vi "Merge.vi"(6 "Conditional Object":refnum<class>, 8 "error in (no error)":errorcluster, 9 "Object B":refnum<class>, 10 "Object A":refnum<class>, 11 "Overwrite A if A equal in":refnum<class "Overwrite A if A equal.lvclass">) -> (0 "error out":errorcluster, 2 "Output Object":refnum<class>, 3 "Overwrite A if A equal out":refnum<class "Overwrite A if A equal.lvclass">)   [LabVIEW 2020, in "Merge Tools.lvlib" / "Overwrite A if A equal.lvclass"]
uses:
  Overwrite A if A equal.lvclass
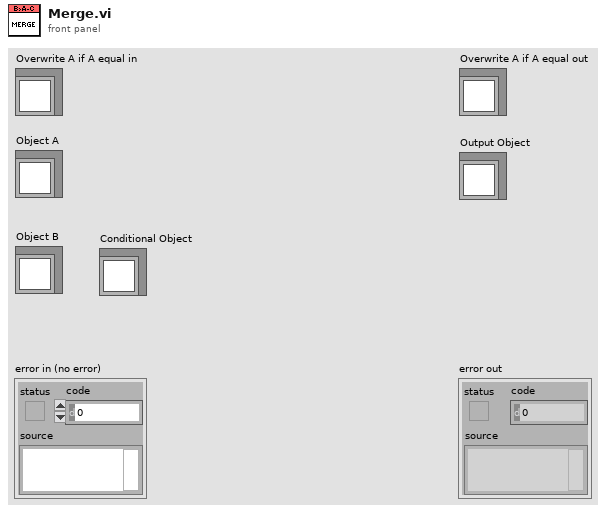
[diagram p1: front panel]
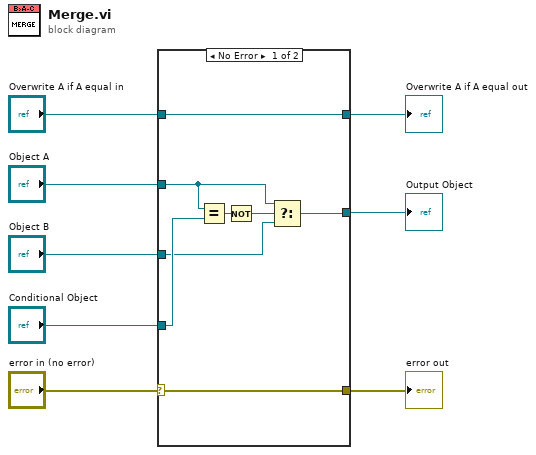
[diagram p0: block diagram]
diagram:
  n1 = case shown="No Error" "error in (no error)" {
    selector: "error in (no error)" -> [w9 w18]
    tunnel: [w9 w18] -> w7
    tunnel: "Overwrite A if A equal in" -> [w10 w17]
    tunnel: [w10 w17] -> w5
    tunnel: "Object A" -> [w13 _]
    tunnel: "Object B" -> [w12 _]
    tunnel: "Conditional Object" -> [w16 _]
    tunnel: [w11 _] -> w1
    frame No Error {
      n2 = Equal?(x=w13, y=w16) -> (x = y?=w15:bool)
      n3 = Not(x=w15) -> (.not. x?=w14:bool)
      n4 = Select(t=w13, s=w14, f=w12) -> (s? t:f=w11:refnum<class>)
    }
    frame Error {
    }
  }
  "error out" <- w7
  "Overwrite A if A equal out" <- w5
  "Output Object" <- w1
